vi "Enclose Objects in Structure.vi"(7 "Top Level Diagram":refnum<vi>, 8 "error in":errorcluster, 10 "Structure Type":T1, 11 "Objects":refnum<vi>[](array[refnum])) -> (0 "error out":errorcluster, 3 "Structure":refnum<vi>)   [LabVIEW 2020, in "Enclose in Structure.lvlib"]
uses:
  Enclose in Structure.lvlib
  Structure Type.ctl
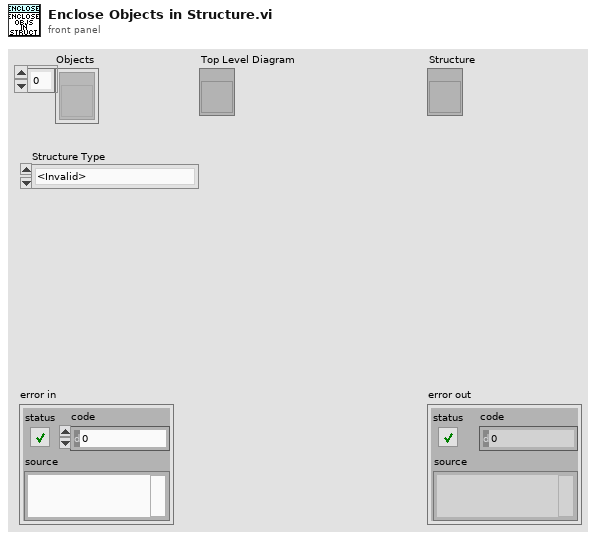
[diagram p1: front panel]
types:
  T1 = typedef "Enclose in Structure.lvlib/Structure Type.ctl" = enum16{"<Invalid>", "For Loop", "While Loop", "Timed Loop", "Timed Sequence", "Case Structure", "Event Structure", "In Place Element Structure", "Flat Sequence", "Diagram Disable Structure", "Conditional Disable Structure", "Type Specialization Structure"}
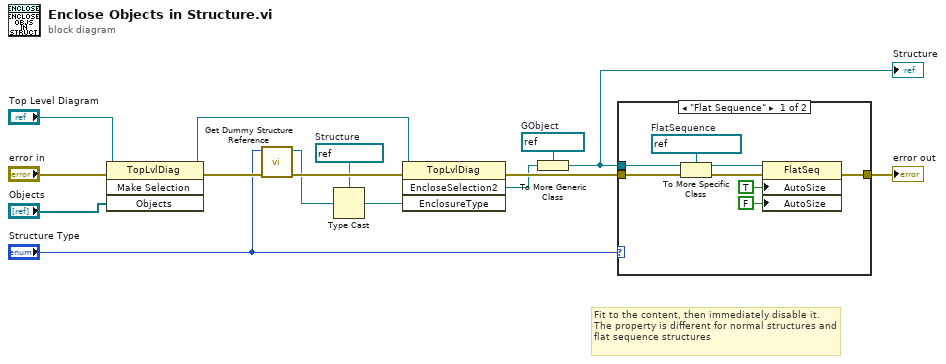
[diagram p0: block diagram]
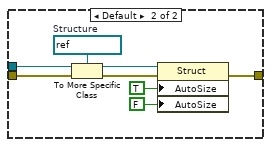
[diagram p2: hidden frame]
diagram:
  w7 = refnum<vi> refnum  # GObject
  w13 = refnum<vi> refnum  # Structure
  # "Fit to the content, then immediately disable it.\nThe property is different for normal structures and flat sequence structures"
  n1 = invoke class="TopLvlDiag" method="Make Selection"(reference="Top Level Diagram", error in="error in", "Objects"="Objects") -> (reference out=w12:refnum<vi>, error out=w3:errorcluster)  [unwired: 1 in, 2 out]
  n2 = call "Get Dummy Structure Reference.vi"("error in"=w3, "Structure Type"="Structure Type") -> ("error out"=w15:errorcluster, "Structure Reference"=w4:refnum<vi>)  [unwired: 8 in]
  n3 = Type Cast(type=w13, x=w4) -> (*(type *) &x=w1:refnum<vi>)
  n4 = invoke class="TopLvlDiag" method="EncloseSelection2"(reference=w12, error in=w15, "EnclosureType"=w1) -> (error out=w14:errorcluster, "EncloseSelection2"=w6:refnum<vi>)  [unwired: 1 in, 2 out]
  n5 = To More Generic Class(target class=w7, reference=w6) -> (generic class reference=w5:refnum<vi>)
  "Structure" <- w5
  n6 = case shown="\"Flat Sequence\"" "Structure Type" {
    tunnel: w14 -> [w23 w24]
    tunnel: w5 -> [w22 w26]
    tunnel: [w21 w31] -> w9
    frame "Flat Sequence" {
      w20 = refnum<vi> refnum  # FlatSequence
      n7 = To More Specific Class(target class=w20, reference=w22, error in=w23) -> (specific class reference=w18:refnum<vi>, error out=w17:errorcluster)
      n8 = property class="FlatSeq"(reference=w18, error in=w17, "AutoSize"=TRUE ("AutoSize To Fit Contents?"), "AutoSize"=FALSE ("AutoSize To Fit Contents?")) -> (error out=w21:errorcluster)  [unwired: 1 out]
    }
    frame Default {
      w28 = refnum<vi> refnum  # Structure
      n9 = To More Specific Class(target class=w28, reference=w26, error in=w24) -> (specific class reference=w27:refnum<vi>, error out=w25:errorcluster)
      n10 = property class="Struct"(reference=w27, error in=w25, "AutoSize"=TRUE ("AutoSize To Fit Contents?"), "AutoSize"=FALSE ("AutoSize To Fit Contents?")) -> (error out=w31:errorcluster)  [unwired: 1 out]
    }
  }
  "error out" <- w9
